vi "Write Value.vi"(8 "error in (no error)":errorcluster, 10 "Data":bool, 11 "Boolean in":refnum<class "Const_Bool.lvclass">) -> (0 "error out":errorcluster, 3 "Boolean out":refnum<class "Const_Bool.lvclass">)   [LabVIEW 2021, in "Const_Bool.lvclass"]
uses:
  Const_Bool.lvclass
  Const_Bool.lvclass/Const_Bool.ctl
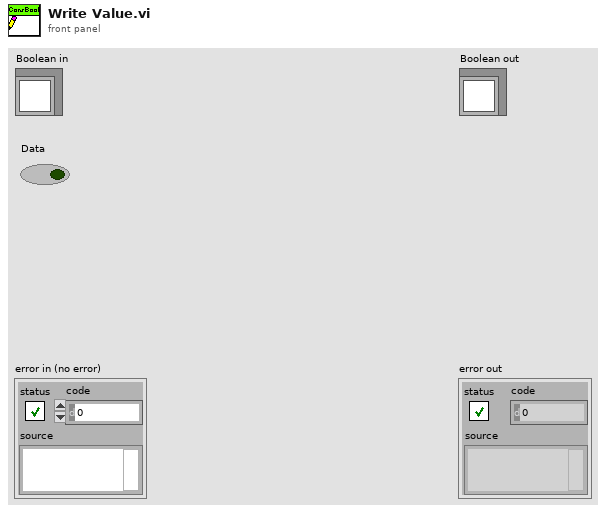
[diagram p1: front panel]
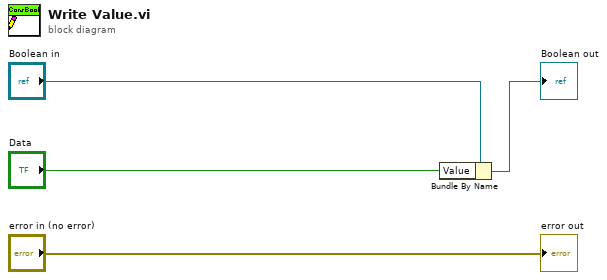
[diagram p0: block diagram]
diagram:
  n1 = Bundle By Name(cluster="Boolean in", "Value"="Data") -> (→"Boolean out":refnum<class "Const_Bool.lvclass">)
  "error out" <- "error in (no error)"
